vi "Construct_multipart_message.vi"(0 "command":T2=enum."configure_rf", 1 "Status":T1, 5 "parameters (JSON)":string="{\"invalid\":1}", 9 "data in":string, 11 "error in (no error)":errorcluster) -> (3 "command_str":string="invalid_command", 4 "Multipart message":string[](array[string]), 14 "Debug info":string, 15 "error out":errorcluster)   [LabVIEW 2019, in "mmW_commands.lvlib"]
uses:
  TypeDefs/commands.ctl
  TypeDefs/response status.ctl
  mmW_commands.lvlib
  TypeDefs/command_types.ctl
panel:
  out "type (none)":string="none"
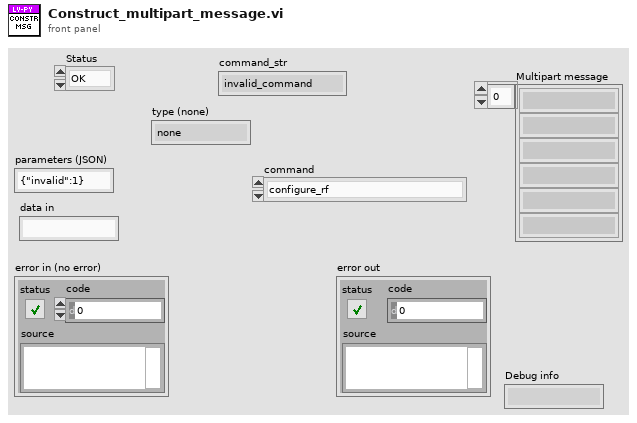
[diagram p1: front panel]
types:
  T1 = typedef "mmW_commands.lvlib/response status.ctl" = enum16{"OK", "Error", "Warning", "Unknown"}
  T2 = typedef "mmW_commands.lvlib/commands.ctl" = enum16{"configure_fs", "configure_rf", "configure_trigger", "equalization_enable", "equalization_start", "lo_sync_enable", "equalization_stop", "get_instrument_status", "get_versions", "initialize_hw", "pop_rx", "set_log_level", "Shutdown", "start", "start_instrument_app", "stop", "trans", "transceive", "trigger_burst", "trigger_sync_enable", "Write TX", "resp_generic", "resp_waveform", "send_trigger", "fetch", "transceive2"}
  T3 = typedef "mmW_commands.lvlib/command_types.ctl" = enum16{"invalid_command", "instrument_control", "environment_control", "response"}
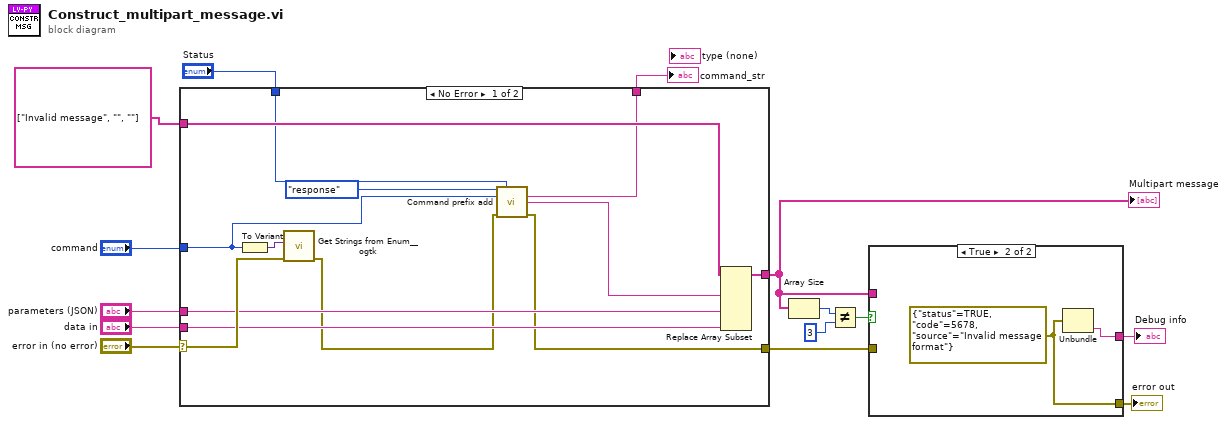
[diagram p0: block diagram]
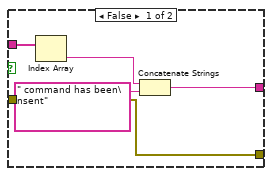
[diagram p2: hidden frame]
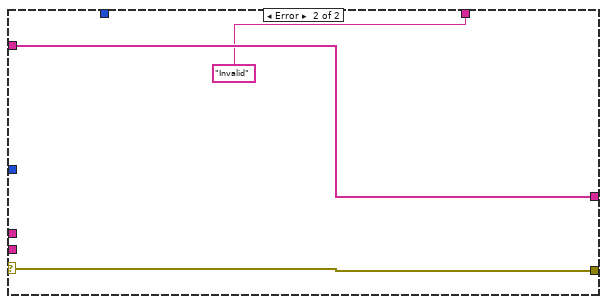
[diagram p3: hidden frame]
diagram:
  n1 = case shown="No Error" "error in (no error)" {
    selector: "error in (no error)" -> [w24 w29]
    tunnel: "parameters (JSON)" -> [w22 _]
    tunnel: [w15 w29] -> w7
    tunnel: [w27 w30] -> w6
    tunnel: string[] ["Invalid message", "", ""] -> [w26 w30]
    tunnel: "command" -> [w19 _]
    tunnel: [w18 "Invalid" ("String Value")] -> w3
    tunnel: "Status" -> [w21 _]
    tunnel: "data in" -> [w23 _]
    frame No Error {
      n2 = To Variant(anything=w19) -> (Variant=w25:variant)
      n3 = call <userlib>:"Get Strings from Enum__ogtk.vi"("error in (no error)"=w24, "Enum"=w25) -> ("error out"=w16:errorcluster)  [unwired: 6 in, 3 out]
      n4 = call "Command prefix add.vi"("Command_Types"=command_types."response", "Status"=w21, "command"=w19, "error in (no error)"=w16) -> ("command str"=w18:string, "prefix+cmd"=w17:string, "error out"=w15:errorcluster)  [unwired: 9 in]
      n5 = Replace Array Subset(array=w26, new element #1=w17, new element #2=w22, new element #3=w23) -> (w27:string[])  [unwired: 3 in]
    }
    frame Error {
    }
  }
  "Multipart message" <- w6
  "command_str" <- w3
  n6 = Array Size(array=w6) -> (size(s)=w11:i32)
  n7 = Not Equal?(x=w11, y=3) -> (x != y?=w9:bool)
  n8 = case shown="True" w9 {
    tunnel: [w35 w37] -> w8
    tunnel: w7 -> [w35 _]
    tunnel: w6 -> [w34 _]
    tunnel: [w31 w36] -> w5
    frame False {
      n9 = Index Array(array=w34) -> (element=w33:string)  [unwired: 1 in]
      n10 = Concatenate Strings(w33, " command has been\nsent" ("string")) -> (w31:string)
    }
    frame True {
      w37 = errorcluster {"status"=TRUE, "code"=5678, "source"="Invalid message format"} ("s? t:f")
      n11 = Unbundle(w37) -> ("source"=w36:string)  [unwired: 2 out]
    }
  }
  "error out" <- w8
  "Debug info" <- w5
